vi "Finalization.vi"(8 "error in":errorcluster) -> (0 "error out":errorcluster)   [LabVIEW 2017]
uses:
  ManageMovableObjects/ManRef_mods.ctl
  Display/Display_mods.ctl
  Spaceship/Spaceship_mods.ctl
  Log/Log_mods.ctl
  ManageMovableObjects/HoldData/HoldData_mods.ctl
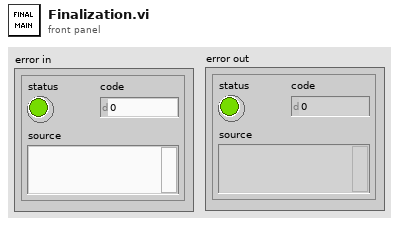
[diagram p1: front panel]
types:
  T1 = typedef "HoldData_mods.ctl" = enum16{"Init", "NewAster", "UpdateAster", "RemoveAster", "GetAsterData", "NewShoot", "UpdateShoot", "RemoveShoot", "GetShootData", "End"}
  T2 = typedef "Log_mods.ctl" = enum16{"Init", "Write", "Clear", "End"}
  T3 = typedef "Spaceship_mods.ctl" = enum16{"Init", "Move", "Rotate", "Translate", "GetData", "End"}
  T4 = typedef "Display_mods.ctl" = enum16{"Init", "GetBase", "AddAster", "UpdateShip", "AddShoot", "DrawAll", "Clear", "Close"}
  T5 = typedef "ManRef_mods.ctl" = enum16{"Init", "NewAster", "MoveAll", "DestroyAster", "NewShoot", "DestroyShot", "CheckColision", "End"}
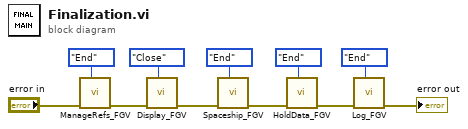
[diagram p0: block diagram]
diagram:
  n1 = call "ManageRefs_FGV.vi"("ManRef_mods"=ManRef_mods."End", "error in"="error in") -> ("error out"=w10:errorcluster)  [unwired: 8 in, 1 out]
  n2 = call "Display_FGV.vi"("Display_mods"=Display_mods."Close", "error in"=w10) -> ("error out"=w7:errorcluster)  [unwired: 8 in, 1 out]
  n3 = call "Spaceship_FGV.vi"("Spaceship_mods"=Spaceship_mods."End", "error in"=w7) -> ("error out"=w2:errorcluster)  [unwired: 8 in, 1 out]
  n4 = call "HoldData_FGV.vi"("HoldData_mods"=HoldData_mods."End", "error in"=w2) -> ("error out"=w1:errorcluster)  [unwired: 8 in, 1 out]
  n5 = call "Log_FGV.vi"("Log_mods"=Log_mods."End", "error in"=w1) -> ("error out"=→"error out":errorcluster)  [unwired: 9 in]
